vi "Initialize.vi"(2 "XRef":refnum<vi>) -> (1 "State Out":T1)   [LabVIEW 2012, in "Foreign Key Sort.xnode"]
uses:
  Foreign Key Sort.xnode
  State.ctl
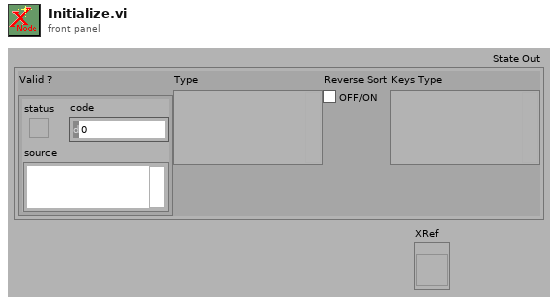
[diagram p1: front panel]
types:
  T1 = typedef "Foreign Key Sort.xnode/State.ctl" = cluster{"Valid ?":errorcluster, "Type":variant, "Reverse Sort":bool, "Keys Type":variant}
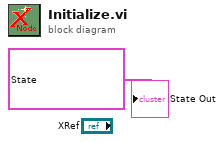
[diagram p0: block diagram]
diagram:
  "State Out" <- T1 {"Valid ?"={"status"=TRUE, "code"=-1, "source"="Initialised"}, "Type"=variant, "Reverse Sort"=FALSE, "Keys Type"=variant} ("State Out")
